vi "Configure Modulation Low Level (PWM Source).vi"(8 "error in":errorcluster, 10 "PWM Source (Internal)":enum16{"Internal", "External"}(ring), 11 "VISA resource name":refnum<visa-resource-name>) -> (0 "error out":errorcluster, 3 "VISA resource name out":refnum<visa-resource-name>)   [LabVIEW 2017, in "Keithley 3390.lvlib"]
doc: "Selects the source of the modulating signal."
uses:
  Keithley 3390.lvlib
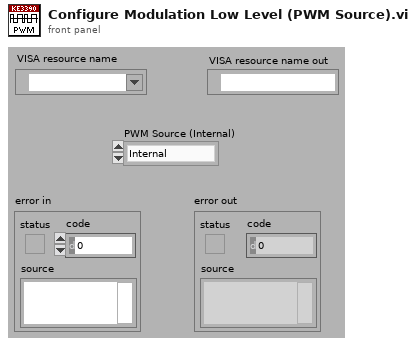
[diagram p1: front panel]
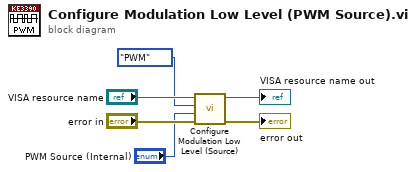
[diagram p0: block diagram]
diagram:
  n1 = call "Configure Modulation Low Level (Source).vi"("error in (no error)"="error in", "Source (Internal)"="PWM Source (Internal)", "Modulation (AM)"=enum16{"AM", "FM", "PM", "FSK", "PWM"}."PWM" ("Modulation (0:AM)"), "VISA resource name"="VISA resource name") -> ("error out"=→"error out":errorcluster, "VISA resource name out"=→"VISA resource name out":refnum<visa-resource-name>)  [unwired: 6 in]
